vi "simplePID Memory Write_FXP.vi"(0 "Memory In":refnum<k21>="Data", 1 "channel (0)":u16, 2 "Input Selector":u16, 11 "state in":T1) -> ()   [LabVIEW 2020]
uses:
  Typedef/niFpgaPID_PIDState_FXP.ctl
  Typedef/niFpgaPID_PIDMemoryItem_FXP.ctl
  <vilib>/rvi/DataTransferAndStorage/Container/Common/niFpgaContainerExecOnDevCompGetState.vi
  <vilib>/rvi/Emulation/niFpgaEmulationIsFPGAContextNoSignature.vi
  <vilib>/rvi/DataTransferAndStorage/Container/Common/niFpgaContainerGetUniqueNameForEmu.vi
  <vilib>/rvi/Emulation/niFpgaProcessEmulError.vi
  <vilib>/rvi/Emulation/niFpgaSctlEmulationGetInTimedLoop.vi
  <vilib>/rvi/errors/nirviReportUnexpectedCaseInternalError (U32).vi
  <vilib>/rvi/Memory/Memory_Emulation/niFpgaMemoryEmulationCacheClearOnFirstRun.vi
  <vilib>/rvi/Memory/Memory_Emulation/nirvimemoryEmulationManagerCache_MakeExclusive.vi
  <vilib>/rvi/Memory/Memory_Emulation/niFpgaMemoryEmulationValidateCache.vi
  <vilib>/rvi/Memory/Memory_Emulation/nirvimemoryEmulationManagerCache_InsertValue.vi
  <vilib>/Utility/error.llb/Clear Errors.vi
  <vilib>/rvi/Memory/Memory_Emulation/nirvimemoryEmulationManagerCache_ReleaseExclusive.vi
  <vilib>/rvi/Memory/Memory_Emulation/nirvimemoryEmulationManagerCache_GetValue.vi
  <vilib>/rvi/Memory/Memory_Emulation/nirvimemoryEmulationManagerCache_SetValue.vi
  <vilib>/rvi/Emulation/niFpgaSctlEmulationResourceMgr.vi
  <vilib>/rvi/DataTransferAndStorage/Container/XNode/niFpgaContainer.xnode
  <vilib>/rvi/Memory/Memory_Emulation/niFpgaMemoryEmulationRefIn.vi
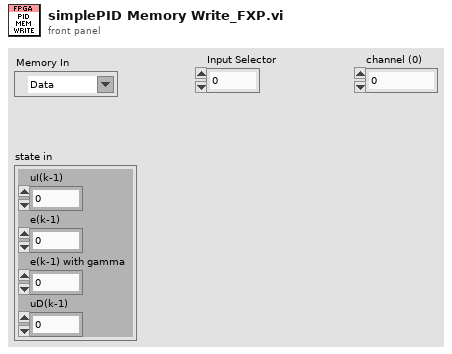
[diagram p1: front panel]
types:
  T1 = typedef "niFpgaPID_PIDState_FXP.ctl" = cluster{"uI(k-1)":fxp<+/-,20,12>, "e(k-1)":fxp<+/-,16,10>, "e(k-1) with gamma":fxp<+/-,16,10>, "uD(k-1)":fxp<+/-,20,12>}
  T2 = typedef "niFpgaPID_PIDMemoryItem_FXP.ctl" = cluster{"data 1":fxp<+/-,20,12>, "data 2":fxp<+/-,16,10>, "data 3":fxp<+/-,16,10>, "data 4":fxp<+/-,20,12>}
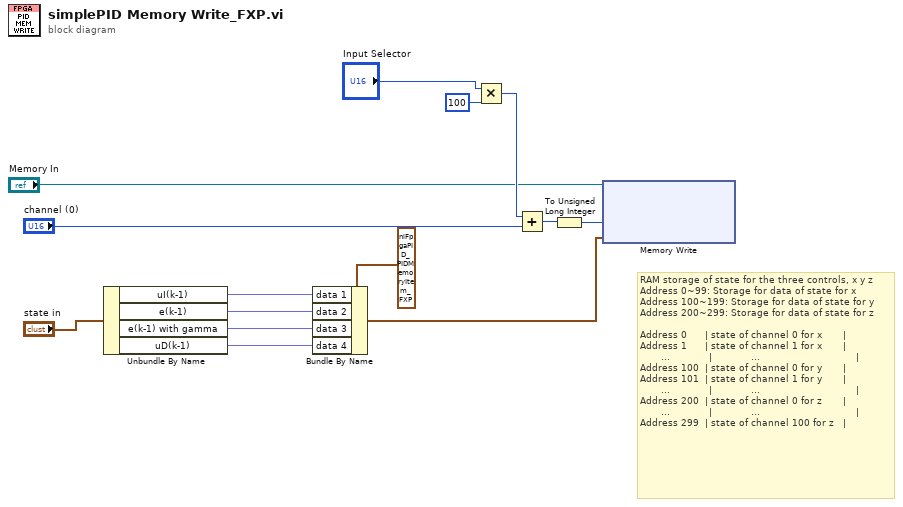
[diagram p0: block diagram]
diagram:
  # "RAM storage of state for the three controls, x y z\nAddress 0~99: Storage for data of state for x\nAddress 100~199: Storage for data of state for y\nAddress 200~299: Storage for data of state for z \n                                                                        \nAddress 0      | state of channel 0 for x       | \nAddress 1      | state of channel 1 for x       | \n       ...             |             ...                                |\nAddress 100  | state of channel 0 for y       | \nAddress 101  | state of channel 1 for y       | \n       ...             |             ...                                |\nAddress 200  | state of channel 0 for z       | \n       ...             |             ...                                |\nAddress 299  | state of channel 100 for z   |"
  n1 = Unbundle By Name("state in") -> ("uI(k-1)"=w13:fxp<+/-,20,12>, "e(k-1)"=w10:fxp<+/-,16,10>, "e(k-1) with gamma"=w11:fxp<+/-,16,10>, "uD(k-1)"=w12:fxp<+/-,20,12>)
  n2 = Bundle By Name(cluster=T2 {"data 1"=0.0, "data 2"=0.0, "data 3"=0.0, "data 4"=0.0} ("PID memory dummy type"), "data 1"=w13, "data 2"=w10, "data 3"=w11, "data 4"=w12) -> (w2:T2)
  n3 = Multiply(x="Input Selector", y=u16 100) -> (x*y=w4:u16)
  n4 = Add(x=w4, y="channel (0)") -> (x+y=w5:u16)
  n5 = To Unsigned Long Integer(number=w5) -> (unsigned 32bit integer=w9:u32)
  n6 = xnode ("Memory Write")("Address"=w9, "Data"=w2, "Memory In"="Memory In") -> ()  [unwired: 1 out]
